vi "Create_Training_Set.vi"() -> ()   [LabVIEW 2009]
uses:
  <vilib>/vision/NI_Vision_Development_Module.lvlib
panel:
  out "Image Sample 2":T1(plugin-control)
  in  "Type of Sample":bool=TRUE
  in  "Not":bool
  in  "Line":bool
  out "Image Sample":T1(plugin-control)
  in  "res/2":i32=4
  in  "stop":bool
  out "Last Mouse Position:All Elements 2":cluster{"X":i32, "Y":i32}={"X"=19, "Y"=30}
  in  "Sample Rate":i32=3
  out "Input Image":T1(plugin-control)
  in  "Iinput File Path":path=path "C:/Documents and Settings/dgrieneisen/My Documents/Robotics/Athena/image2004.jpg"
  out "Output Image":T1(plugin-control)
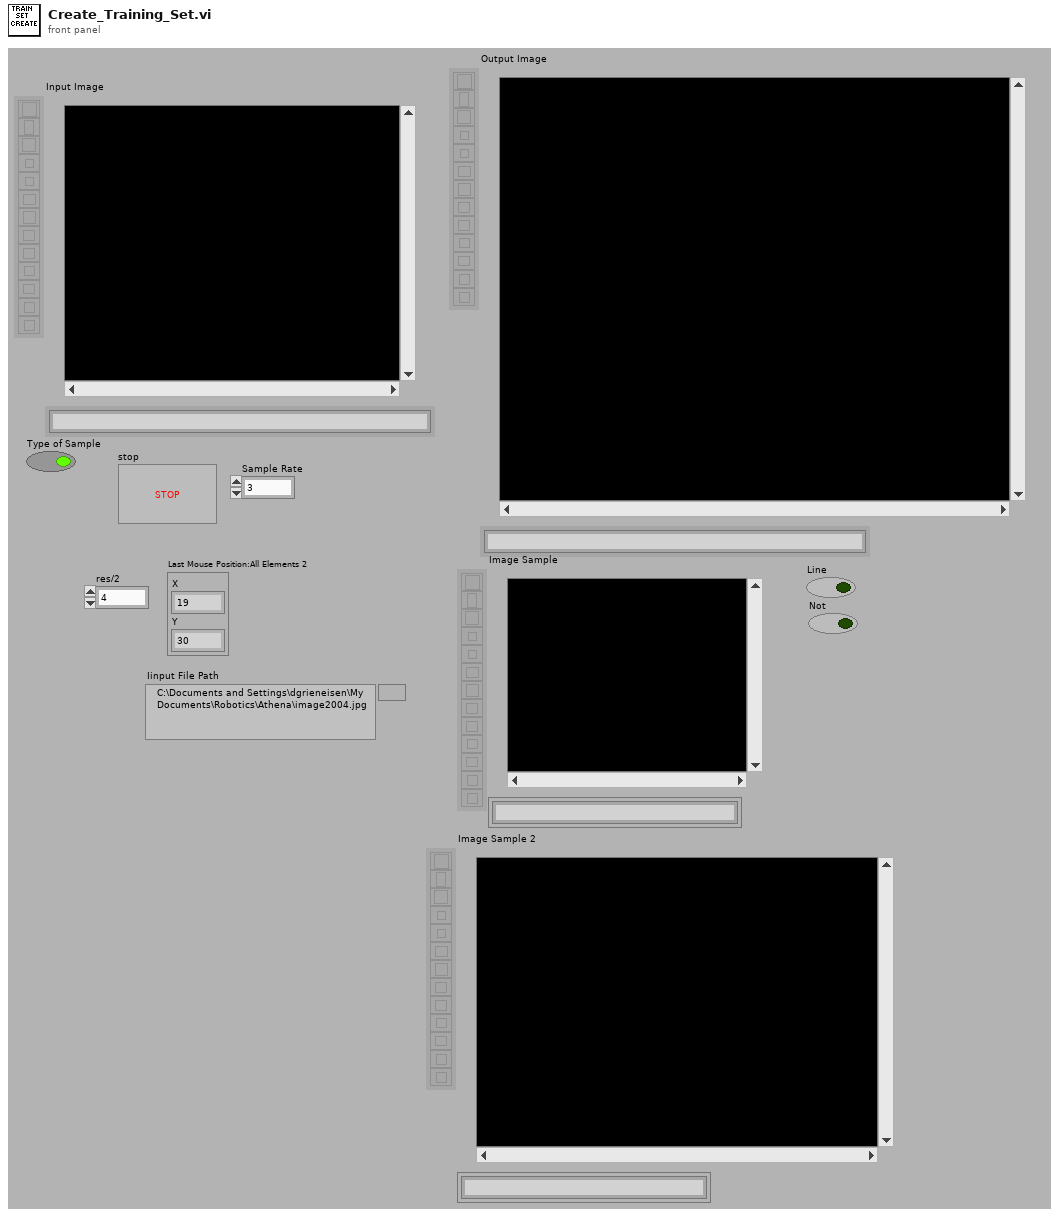
[diagram p1: front panel]
types:
  T1 = typedef "IMAQ Image.ctl" = refnum<image>
  T2 = typedef "Image Type" = u32
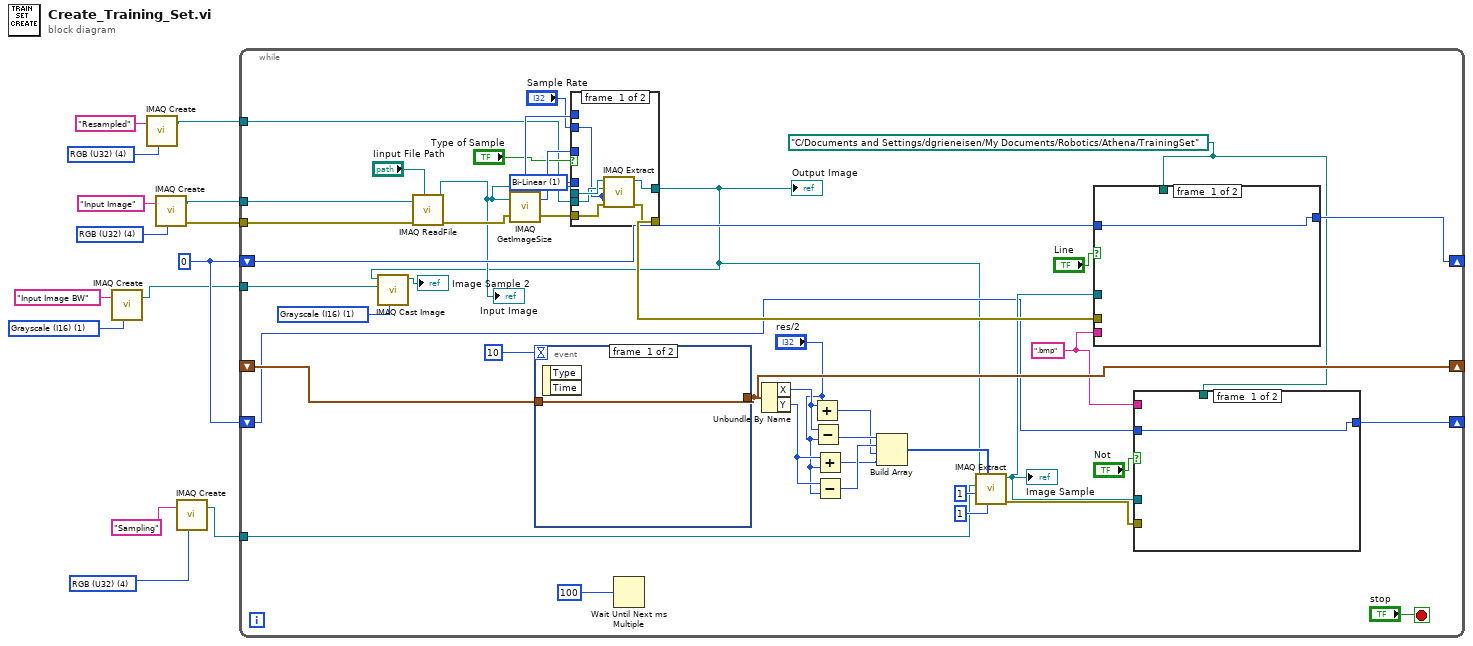
[diagram p0: block diagram]
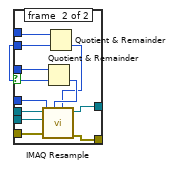
[diagram p2: hidden frame]
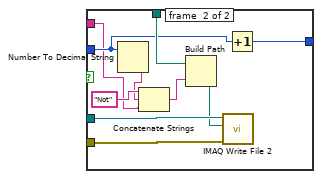
[diagram p3: hidden frame]
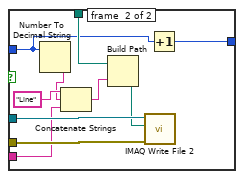
[diagram p4: hidden frame]
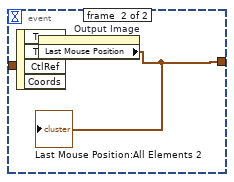
[diagram p5: hidden frame]
diagram:
  w2 = T2 1 items=["Grayscale (U8)", "Grayscale (I16)", "Grayscale (SGL)", "Complex (CSG)", "RGB (U32)", "HSL (U32)", "RGB (U64)", "Grayscale (U16)"] ("Image Type")
  w4 = 0
  w6 = T2 4 items=["Grayscale (U8)", "Grayscale (I16)", "Grayscale (SGL)", "Complex (CSG)", "RGB (U32)", "HSL (U32)", "RGB (U64)", "Grayscale (U16)"] ("Image Type")
  w14 = T2 4 items=["Grayscale (U8)", "Grayscale (I16)", "Grayscale (SGL)", "Complex (CSG)", "RGB (U32)", "HSL (U32)", "RGB (U64)", "Grayscale (U16)"] ("Image Type")
  w12 = T2 4 items=["Grayscale (U8)", "Grayscale (I16)", "Grayscale (SGL)", "Complex (CSG)", "RGB (U32)", "HSL (U32)", "RGB (U64)", "Grayscale (U16)"] ("Image Type")
  n1 = call "IMAQ Create"("Image Name"="Input Image BW", "Image Type"=w2) -> ("New Image"=w1:T1)  [unwired: 2 in, 2 out]
  n2 = call "IMAQ Create"("Image Name"="Resampled", "Image Type"=w14) -> ("New Image"=w8:T1)  [unwired: 2 in, 2 out]
  n3 = call "IMAQ Create"("Image Name"="Input Image", "Image Type"=w12) -> ("New Image"=w10:T1, "error out"=w9:errorcluster)  [unwired: 2 in, 1 out]
  n4 = call "IMAQ Create"("Image Name"="Sampling", "Image Type"=w6) -> ("New Image"=w5:T1)  [unwired: 2 in, 2 out]
  n5 = while {
    shift-right: [w49] -> _
    shift-left: _ -> [w48]
    tunnel: w10 -> [w44]
    tunnel: w9 -> [w43]
    tunnel: w8 -> [w21]
    tunnel: w5 -> [w42]
    shift-right: [w31] -> _
    shift-left: w4 -> [w32]
    shift-right: [w26] -> _
    shift-left: w4 -> [w25]
    tunnel: w1 -> [w19]
    stop <- "stop" stop-if-true
    w18 = T2 1 items=["Grayscale (U8)", "Grayscale (I16)", "Grayscale (SGL)", "Complex (CSG)", "RGB (U32)", "HSL (U32)", "RGB (U64)", "Grayscale (U16)"] ("Image Type")
    w23 = u32 1 items=["Zero Order", "Bi-Linear", "Quadratic", "Cubic Spline"] ("Interpolation Type")
    w24 = ".bmp"
    w27 = path "C:/Documents and Settings/dgrieneisen/My Documents/Robotics/Athena/TrainingSet"
    n6 = call "IMAQ ReadFile"("File Path"="Iinput File Path", "error in (no error)"=w43, "Image"=w44) -> ("error out"=w56:errorcluster, "Image Out"=w16:T1)  [unwired: 4 in, 3 out]
    "Input Image" <- w16
    n7 = call "IMAQ GetImageSize"("Image"=w16, "error in (no error)"=w56) -> ("Y Resolution"=w53:i32, "X Resolution"=w54:i32, "error out"=w55:errorcluster)  [unwired: 2 in]
    n8 = event shown="[1] \"Output Image\": Mouse Down" {
      selector: _ -> [_ _]
      dyn-events: _ -> [_ _]
      timeout: 10 -> [_ _]
      tunnel: [w97 w98] -> w49
      tunnel: w48 -> [w97 _]
      event #0 {
        n9 = event-data() -> ()  [unwired: 1 in, 2 out]
      }
      event #1 {
        n10 = event-data() -> ()  [unwired: 1 in, 4 out]
        n11 = property on="Output Image" class="ImageControl"() -> ("Last Mouse Position"=w98:cluster{"X":i32, "Y":i32})  [unwired: 2 in, 2 out]
        "Last Mouse Position:All Elements 2" <- w98
      }
    }
    n12 = case shown="False" "Type of Sample" {
      tunnel: w16 -> [w63 w74]
      tunnel: w55 -> [w61 w73]
      tunnel: w54 -> [_ w72]
      tunnel: w53 -> [_ w71]
      tunnel: "Sample Rate" -> [w59 w68]
      tunnel: w21 -> [w60 w67]
      tunnel: [w58 w66] -> w15
      tunnel: [w62 w65] -> w33
      tunnel: w23 -> [_ w64]
      frame #0 {
        n13 = call "IMAQ Extract"("Y Step Size"=w59, "error in (no error)"=w61, "X Step Size"=w59, "Image Dst"=w60, "Image Src"=w63) -> ("error out"=w62:errorcluster, "Image Dst Out"=w58:T1)  [unwired: 1 in, 4 out]
      }
      frame #1 {
        n14 = Quotient & Remainder(x=w71, y=w68) -> (floor(x/y)=w70:i32)  [unwired: 1 out]
        n15 = Quotient & Remainder(x=w72, y=w68) -> (floor(x/y)=w69:i32)  [unwired: 1 out]
        n16 = call "IMAQ Resample"("X Resolution"=w69, "Y Resolution"=w70, "error in (no error)"=w73, "Interpolation Type"=w64, "Image Dst"=w67, "Image Src"=w74) -> ("error out"=w65:errorcluster, "Image Dst Out"=w66:T1)  [unwired: 4 in]
      }
    }
    "Output Image" <- w15
    n17 = call "IMAQ Cast Image"("Image Type"=w18, "Image Dst"=w19, "Image Src"=w15) -> ("Image Dst Out"=→"Image Sample 2":T1)  [unwired: 7 in, 1 out]
    n18 = Wait Until Next ms Multiple(millisecond multiple=u32 100) -> ()  [unwired: 1 out]
    n19 = Unbundle By Name(w49) -> ("X"=w40:i32, "Y"=w41:i32)
    n20 = Add(x=w40, y="res/2") -> (x+y=w35:i32)
    n21 = Subtract(x=w40, y="res/2") -> (x-y=w38:i32)
    n22 = Add(x=w41, y="res/2") -> (x+y=w36:i32)
    n23 = Subtract(x=w41, y="res/2") -> (x-y=w37:i32)
    n24 = Build Array(w38, w37, w35, w36) -> (w39:i32[])
    n25 = call "IMAQ Extract"("Y Step Size"=1, "Optional Rectangle"=w39, "X Step Size"=1, "Image Dst"=w42, "Image Src"=w15) -> ("error out"=w28:errorcluster, "Image Dst Out"=w29:T1)  [unwired: 1 in, 4 out]
    "Image Sample" <- w29
    n26 = case shown="True" "Line" {
      tunnel: w29 -> [_ w96]
      tunnel: w33 -> [_ w95]
      tunnel: w27 -> [_ w94]
      tunnel: w32 -> [w86 w92]
      tunnel: [w86 w93] -> w31
      tunnel: w24 -> [_ w87]
      frame #0 {
      }
      frame #1 {
        n27 = Number To Decimal String(number=w92) -> (decimal integer string=w88:string)  [unwired: 1 in]
        n28 = Concatenate Strings("Line", w88, w87) -> (w90:string)
        n29 = Build Path(base path=w94, name or relative path=w90) -> (appended path=w91:path)
        n30 = call-poly "IMAQ Write File 2"("error in (no error)"=w95, "File Path"=w91, "Image"=w96) -> ()  [unwired: 7 in, 2 out]
        n31 = Increment(x=w92) -> (x+1=w93:i32)
      }
    }
    n32 = case shown="True" "Not" {
      tunnel: w29 -> [_ w85]
      tunnel: w28 -> [_ w84]
      tunnel: w27 -> [_ w83]
      tunnel: w25 -> [w75 w81]
      tunnel: [w75 w82] -> w26
      tunnel: w24 -> [_ w76]
      frame #0 {
      }
      frame #1 {
        n33 = Number To Decimal String(number=w81) -> (decimal integer string=w77:string)  [unwired: 1 in]
        n34 = Concatenate Strings("Not", w77, w76) -> (w79:string)
        n35 = Build Path(base path=w83, name or relative path=w79) -> (appended path=w80:path)
        n36 = call-poly "IMAQ Write File 2"("error in (no error)"=w84, "File Path"=w80, "Image"=w85) -> ()  [unwired: 7 in, 2 out]
        n37 = Increment(x=w81) -> (x+1=w82:i32)
      }
    }
  }
